vi "drivetrain.vi"() -> ()   [LabVIEW 2011]
uses:
  dashboard/dashboard_data_drivetrain.ctl
  gear_shift_state.ctl
  gear_internal_shift_state.ctl
  signals/Signal.ctl
  drivetrain_drive_mode.ctl
  drivetrain_globals.vi
panel:
  in  "Boolean":bool
  out "Angle":dbl
  # "Drivetrain system"
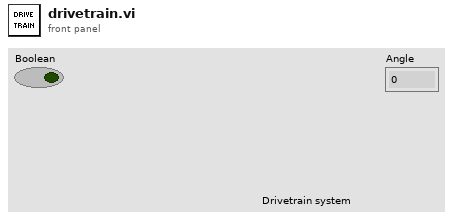
[diagram p1: front panel]
types:
  T1 = typedef "WPI_RobotDriveDevRef.ctl" = cluster{"DevStatus":errorcluster, "Motors[]":T2[], "Square Inputs":bool, "Max Output":dbl}
  T2 = typedef "WPI_MotorControlDeviceRef.ctl" = cluster{"DeviceStatus":errorcluster, "Type":enum16{"PWM", "CAN"}, "PWM":cluster{"Digital Module":T3, "PWM Channel":T4, "DeadBand":T5}, "CAN":cluster{"Device Number":u8, "Control Mode":T6, "Semaphore":T7, "Max Vout":dbl}, "Invert":bool, "TransformRef":T8, "InvTransformRef":T8}
  T3 = typedef "FPGA_TypedefDigitalModule.ctl" = enum16{"Digital Module 1", "Digital Module 2"}
  T4 = typedef "FPGA_DIOPWMChannel.ctl" = enum8{"PWM 1", "PWM 2", "PWM 3", "PWM 4", "PWM 5", "PWM 6", "PWM 7", "PWM 8", "PWM 9", "PWM 10", "Invalid"}
  T5 = typedef "WPI_PWMDeadband.ctl" = cluster{"Name":string, "maxPositivePwm":i32, "minPositivePwm":i32, "centerPwm":i32, "maxNegativePwm":i32, "minNegativePwm":i32, "angularRange":u16}
  T6 = typedef "WPI_CANJaguar_ControlMode.ctl" = enum8{"Percent VBus", "Current", "Speed", "Position", "Voltage"}
  T7 = typedef "Semaphore RefNum" = refnum<k1>
  T8 = typedef "WPI_PWMTransform_ConPane.ctl" = refnum<vi>
  T9 = typedef "WPI_ServoDeviceRef.ctl" = cluster{"DeviceStatus":errorcluster, "Digital Module":T3, "PWM Channel":T4, "DeadBand":T5}
  T10 = typedef "WPI_GyroDevRef.ctl" = cluster{"DevStatus":errorcluster, "Analog Module":T11, "Analog Channel":T12, "Offset":dbl, "Gain (VoltsPerDegree/Second)":dbl}
  T11 = typedef "FPGA_TypedefAnalogModule.ctl" = enum16{"Analog Module 1", "Analog Module 2"}
  T12 = typedef "FPGA_AIChannel.ctl" = enum8{"AI 1", "AI 2", "AI 3", "AI 4", "AI 5", "AI 6", "AI 7", "AI 8", "Invalid"}
  T13 = typedef "dashboard_data_drivetrain.ctl" = cluster{"left":cluster{"request":dbl, "enc_speed":dbl}, "right":cluster{"request":dbl, "enc_speed":dbl}, "gear shift state":T14, "gear shift internal state":T15}
  T14 = typedef "gear_shift_state.ctl" = enum16{"low", "high"}
  T15 = typedef "gear_internal_shift_state.ctl" = enum16{"low", "high", "low_peak", "high_peak"}
  T16 = enum16{"push_data", "write_joe_johnson", "write_roller", "write_drivetrain", "write_gun_fast", "write_gun_slow"}
  T17 = typedef "Signal.ctl" = enum16{"SIGFIRE", "SIGSTOPSCRIPT", "SIGSTARTGUN", "SIGSTOPGUN", "SIGDISABLED", "SIGENABLED", "SIGUDPTIMEOUT", "SIGNEWVISION_REMOTE", "SIGNEWVISION_LOCAL", "SIGSHOTFIRED", "SIGDOTRACK", "SIGDONTTRACK"}
  T18 = typedef "drivetrain_drive_mode.ctl" = enum16{"open loop", "closed loop"}
  T19 = typedef "drivetrain_drive_write_thread.ctl" = enum16{"Teleop", "Script Engine - Autonomous", "Script Engine - Sequence"}
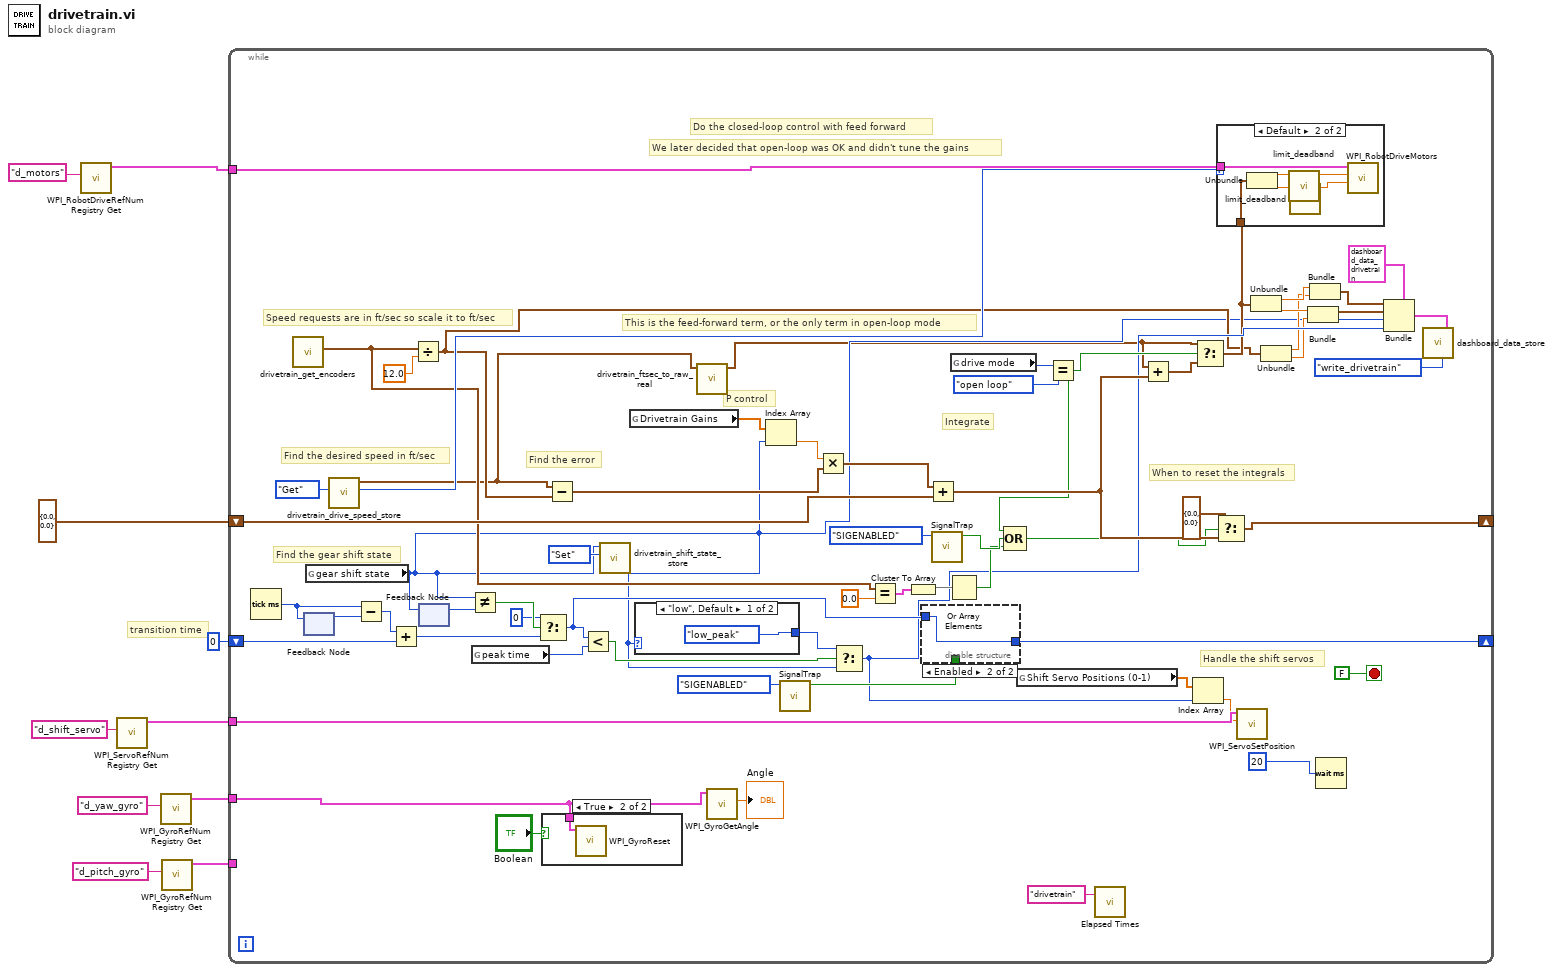
[diagram p0: block diagram]
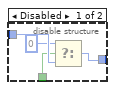
[diagram p2: hidden frame]
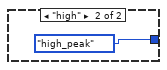
[diagram p4: hidden frame]
diagram:
  # "transition time"
  n1 = call <vilib>:"WPI_RobotDriveRefNum Registry Get.vi"("refnum name"="d_motors") -> ("RobotDriveDevRef"=w9:T1)  [unwired: 9 in, 1 out]
  n2 = call <vilib>:"WPI_ServoRefNum Registry Get.vi"("refnum name"="d_shift_servo") -> ("ServoDeviceRef"=w6:T9)  [unwired: 9 in, 1 out]
  n3 = call <vilib>:"WPI_GyroRefNum Registry Get.vi"("refnum name"="d_yaw_gyro") -> ("GyroDevRef"=w3:T10)  [unwired: 9 in, 1 out]
  n4 = call <vilib>:"WPI_GyroRefNum Registry Get.vi"("refnum name"="d_pitch_gyro") -> ("GyroDevRef"=w2:T10)  [unwired: 9 in, 1 out]
  n5 = while {
    tunnel: w9 -> [w73]
    shift-right: [w64] -> _
    shift-left: cluster{"Left":dbl, "Right":dbl} {"Left"=0.0, "Right"=0.0} -> [w66]
    tunnel: w6 -> [w57]
    tunnel: w3 -> [w32]
    tunnel: w2 -> [_]
    shift-right: [w28] -> _
    shift-left: u32 0 ("t") -> [w38]
    stop <- FALSE stop-if-true
    # "We later decided that open-loop was OK and didn't tune the gains"
    # "When to reset the integrals"
    # "Handle the shift servos"
    # "Integrate"
    # "P control"
    # "Find the error"
    # "Find the desired speed in ft/sec"
    # "This is the feed-forward term, or the only term in open-loop mode"
    # "Find the gear shift state"
    # "Speed requests are in ft/sec so scale it to ft/sec"
    # "Do the closed-loop control with feed forward"
    n6 = Tick Count (ms)() -> (millisecond timer value=w41:u32)
    n7 = call "drivetrain_get_encoders.vi"() -> ("Velocity (in/sec)"=w44:cluster{"Left":dbl, "Right":dbl})  [unwired: 9 in, 2 out]
    n8 = feedback-in #1(w41) -> ()
    n9 = feedback #1() -> (w40:u32)  [unwired: 1 in]
    n10 = global read "drivetrain_globals.vi" "gear shift state"() -> (w13:T14)
    n11 = call "drivetrain_drive_speed_store.vi"("data_store_mode"=enum16{"Set", "Get"}."Get") -> ("lock thread"=w45:T19, "drive data out"=w12:cluster{"Left":dbl, "Right":dbl})  [unwired: 9 in]
    n12 = Subtract(x=w41, y=w40) -> (x-y=w39:u32)
    n13 = Add(x=w39, y=w38) -> (x+y=w37:u32)
    n14 = Divide(x=w44, y=12.0) -> (x/y=w15:cluster{"Left":dbl, "Right":dbl})
    n15 = feedback-in #2(w13) -> ()
    n16 = feedback #2() -> (w43:T14)  [unwired: 1 in]
    n17 = Not Equal?(x=w13, y=w43) -> (x != y?=w42:bool)
    n18 = global read "drivetrain_globals.vi" "peak time"() -> (w35:u32)
    n19 = Select(t=u32 0, s=w42, f=w37) -> (s? t:f=w29:u32)
    n20 = case shown="True" "Boolean" {
      tunnel: w32 -> [_ w80]
      frame False {
      }
      frame True {
        n21 = call <vilib>:"WPI_GyroReset.vi"("GyroDevRef"=w80) -> ()  [unwired: 9 in, 2 out]
      }
    }
    n22 = Subtract(x=w12, y=w15) -> (x-y=w68:cluster{"Left":dbl, "Right":dbl})
    n23 = Less?(x=w29, y=w35) -> (x < y?=w33:bool)
    n24 = call "drivetrain_shift_state_store.vi"("data_store_mode"=enum16{"Set", "Get"}."Set", "gear shift state"=w13) -> ()  [unwired: 9 in, 1 out]
    n25 = global read "drivetrain_globals.vi" "Drivetrain Gains"() -> (w70:dbl[])
    n26 = case shown="\"low\", Default" w13 {
      tunnel: [gear_internal_shift_state."low_peak" ("gear shift state") gear_internal_shift_state."high_peak" ("gear shift state")] -> w34
      frame "low", Default {
      }
      frame "high" {
      }
    }
    n27 = call "drivetrain_ftsec_to_raw_real.vi"("Drive Data"=w12) -> ("Drive Data Out"=w11:cluster{"Left":dbl, "Right":dbl})  [unwired: 10 in]
    n28 = call <vilib>:"WPI_GyroGetAngle.vi"("GyroDevRef"=w32) -> ("Angle"=→"Angle":dbl)  [unwired: 7 in, 3 out]
    n29 = Index Array(array=w70, index=w13) -> (element=w69:dbl)
    n30 = call "SignalTrap.vi"("Signal"=Signal."SIGENABLED") -> ("Trapped Signal"=w27:bool)  [unwired: 10 in]
    n31 = Multiply(x=w69, y=w68) -> (x*y=w67:cluster{"Left":dbl, "Right":dbl})
    n32 = Select(t=w34, s=w33, f=w13) -> (s? t:f=w23:T15)
    n33 = Equal?(x=w44, y=0.0) -> (x = y?=w50:cluster{"Left":bool, "Right":bool})
    n34 = Cluster To Array(cluster=w50) -> (array=w49:bool[])
    n35 = disable-structure shown="Enabled" {
      disable-tunnel: w29 -> [w78 w79]
      disable-tunnel: [w77 w79] -> w28
      disable-tunnel: w27 -> [w75 _]
      frame Disabled {
        n36 = Select(t=u32 0, s=w75, f=w78) -> (s? t:f=w77:u32)
      }
      frame Enabled {
      }
    }
    n37 = Add(x=w67, y=w66) -> (x+y=w63:cluster{"Left":dbl, "Right":dbl})
    n38 = call "SignalTrap.vi"("Signal"=Signal."SIGENABLED") -> ("Trapped Signal"=w52:bool)  [unwired: 10 in]
    n39 = Or Array Elements(Boolean array=w49) -> (logical OR=w48:bool)
    n40 = global read "drivetrain_globals.vi" "drive mode"() -> (w61:T18)
    n41 = global read "drivetrain_globals.vi" "Shift Servo Positions (0-1)"() -> (w56:dbl[])
    n42 = Equal?(x=w61, y=drivetrain_drive_mode."open loop") -> (x = y?=w58:bool)
    n43 = Compound Arithmetic op=OR(w58, w52, w48) -> (w59:bool)
    n44 = call "Elapsed Times.vi"("Call Name"="drivetrain") -> ()  [unwired: 2 in, 1 out]
    n45 = Add(x=w11, y=w63) -> (x+y=w62:cluster{"Left":dbl, "Right":dbl})
    n46 = Index Array(array=w56, index=w23) -> (element=w55:dbl)
    n47 = Select(t=w11, s=w58, f=w62) -> (s? t:f=w22:cluster{"Left":dbl, "Right":dbl})
    n48 = Select(t=cluster{"Left":dbl, "Right":dbl} {"Left"=0.0, "Right"=0.0}, s=w59, f=w63) -> (s? t:f=w64:cluster{"Left":dbl, "Right":dbl})
    n49 = case shown="Default" w45 {
      tunnel: w73 -> [_ w88]
      tunnel: w22 -> [_ w87]
      frame "Script Engine - Autonomous" {
      }
      frame Default {
        n50 = Unbundle(w87) -> ("Left"=w86:dbl, "Right"=w84:dbl)
        n51 = call "limit_deadband.vi"("Val"=w86) -> ("Val Out"=w85:dbl)  [unwired: 10 in]
        n52 = call "limit_deadband.vi"("Val"=w84) -> ("Val Out"=w83:dbl)  [unwired: 10 in]
        n53 = call <vilib>:"WPI_RobotDriveMotors.vi"("RightSpeed"=w83, "LeftSpeed"=w85, "RobotDriveDevRef"=w88) -> ()  [unwired: 7 in, 2 out]
      }
    }
    n54 = call <vilib>:"WPI_ServoSetPosition.vi"("Position"=w55, "ServoDeviceRef"=w57) -> ()  [unwired: 8 in, 2 out]
    n55 = Unbundle(w22) -> ("Left"=w21:dbl, "Right"=w18:dbl)
    n56 = Unbundle(w15) -> ("Left"=w17:dbl, "Right"=w16:dbl)
    n57 = Bundle("Right"=w18, "Right"=w16) -> (w19:cluster{"Right":dbl, "Right":dbl})  [unwired: 1 in]
    n58 = Bundle("Left"=w21, "Left"=w17) -> (w20:cluster{"Left":dbl, "Left":dbl})  [unwired: 1 in]
    n59 = Wait (ms)(milliseconds to wait=u32 20 ("millisecond multiple")) -> ()  [unwired: 1 out]
    n60 = Bundle(cluster=T13 {"left"={"request"=0.0, "enc_speed"=0.0}, "right"={"request"=0.0, "enc_speed"=0.0}, "gear shift state"=enum."low", "gear shift internal state"=enum."low"} ("drivetrain_data"), "left"=w20, "right"=w19, "gear shift state"=w13, "gear shift internal state"=w23) -> (w24:T13)
    n61 = call "dashboard_data_store.vi"("mode"=T16."write_drivetrain", "drivetrain_data"=w24) -> ()  [unwired: 10 in]
  }
